vi "User Interface Test.vi"() -> ()   [LabVIEW 2017, in "DSF Core.lvlib"]
uses:
  DSF Core.lvlib
  Typedefs/DSF Version Info.ctl
  Classes/User Interface/Core/Core User Interfaces.lvclass
  C:/Git/DSF/Core/Classes/Component User Interface/Component User Interfaces.lvclass
  Classes/User Interface Handler/User Interface Handler.lvclass
  Classes/User Interface/User Interface.lvclass
  Classes/Component User Interface/Component User Interfaces.lvclass
panel:
  out "settings":cluster{"key":string, "value":string}[](array[cluster])
  in  "stop":bool
  in  "Type":T1(ring)
  out "data format":T2
  in  "stop subpanel":bool
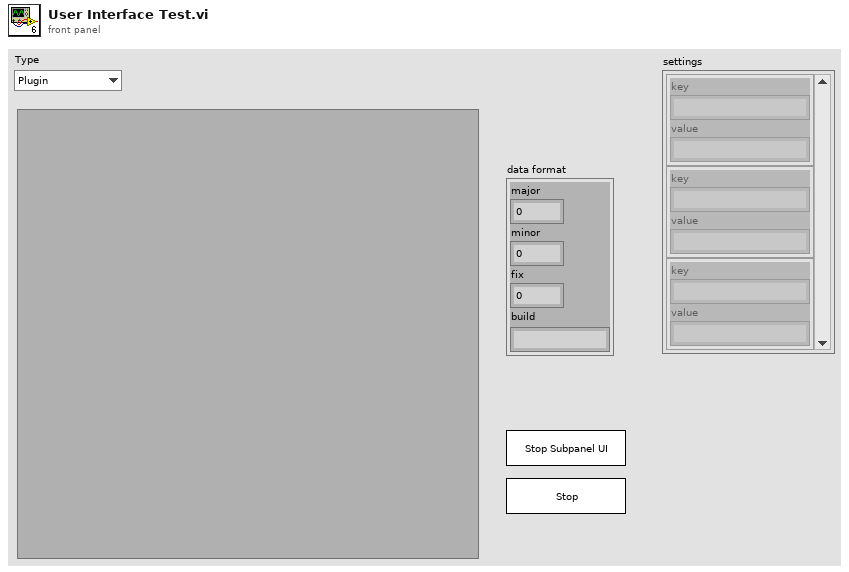
[diagram p1: front panel]
types:
  T1 = enum16{"Plugin", "Thread", "Group", "Transfer", "Channel"}
  T2 = typedef "DSF Core.lvlib/DSF Version Info.ctl" = cluster{"major":u32, "minor":u32, "fix":u32, "build":string}
  T3 = typedef "DSF Core.lvlib/User Interface Handler.lvclass/User Interface Ref.ctl" = refnum<vi>
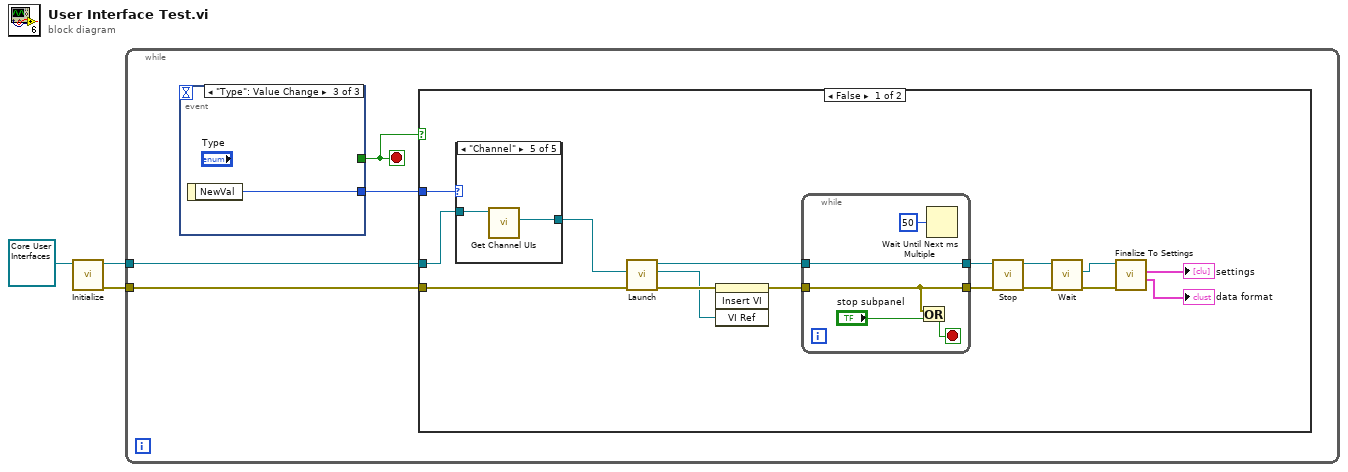
[diagram p0: block diagram]
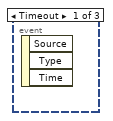
[diagram p2: hidden frame]
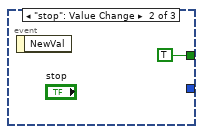
[diagram p3: hidden frame]
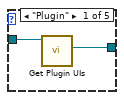
[diagram p4: hidden frame]
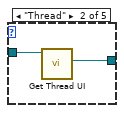
[diagram p5: hidden frame]
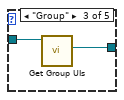
[diagram p6: hidden frame]
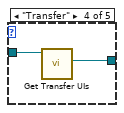
[diagram p7: hidden frame]
diagram:
  n1 = call-dynamic "Initialize.vi"("Component UI in"=refnum<class "Core User Interfaces.lvclass"> refnum ("DSF Core.lvlib:Core Configuration UI.lvclass")) -> ("error out"=w1:errorcluster, "Component UI out"=w2:refnum<class "Core User Interfaces.lvclass">)  [unwired: 9 in]
  n2 = while {
    tunnel: w2 -> [w7]
    tunnel: w1 -> [w4]
    stop <- w6 stop-if-true
    n3 = event shown="[2] \"Type\": Value Change" {
      selector: _ -> [_ _ _]
      dyn-events: _ -> [_ _ _]
      timeout: _ -> [_ _ _]
      tunnel: [_ TRUE _] -> w6
      tunnel: [_ _ w9] -> w5
      event Timeout {
        n4 = event-data() -> ()  [unwired: 1 in, 3 out]
      }
      event "stop": Value Change {
        n5 = event-data() -> ()  [unwired: 1 in, 1 out]
      }
      event "Type": Value Change {
        n6 = event-data() -> ("NewVal"=w9:T1)  [unwired: 1 in]
      }
    }
    n7 = case shown="False" w6 {
      tunnel: w7 -> [w17 _]
      tunnel: w5 -> [w18 _]
      tunnel: w4 -> [w15 _]
      frame False {
        n8 = case shown="\"Channel\"" w18 {
          tunnel: w17 -> [w32 w34 w36 w38 w40]
          tunnel: [w31 w33 w35 w37 w39] -> w11
          frame "Plugin" {
            n9 = call "Get Plugin UIs.vi"("Component UI in"=w32) -> ("Plugin Settings UI"=w31:refnum<class "User Interface.lvclass">)  [unwired: 8 in, 2 out]
          }
          frame "Thread" {
            n10 = call "Get Thread UI.vi"("Component UI in"=w34) -> ("Thread Settings UI"=w33:refnum<class "User Interface.lvclass">)  [unwired: 8 in, 2 out]
          }
          frame "Group" {
            n11 = call "Get Group UIs.vi"("Component UI in"=w36) -> ("Rx Group UI"=w35:refnum<class "User Interface.lvclass">)  [unwired: 7 in, 3 out]
          }
          frame "Transfer" {
            n12 = call "Get Transfer UIs.vi"("Component UI in"=w38) -> ("Rx Transfer UI"=w37:refnum<class "User Interface.lvclass">)  [unwired: 7 in, 3 out]
          }
          frame "Channel" {
            n13 = call "Get Channel UIs.vi"("Component UI in"=w40) -> ("Rx Channel UI"=w39:refnum<class "User Interface.lvclass">)  [unwired: 7 in, 3 out]
          }
        }
        n14 = call "Launch.vi"("error in (no error)"=w15, "User Interface"=w11) -> ("error out"=w14:errorcluster, "active vi"=w13:T3, "User Interface Handler out"=w12:refnum<class "User Interface Handler.lvclass">)  [unwired: 7 in]
        n15 = invoke on="Sub Panel" class="SubPnl" method="Insert VI"(error in=w14, "VI Ref"=w13) -> (error out=w25:errorcluster)  [unwired: 2 in, 3 out]
        n16 = while {
          tunnel: w25 -> [w29]
          tunnel: [w29] -> w23
          tunnel: w12 -> [w26]
          tunnel: [w26] -> w24
          stop <- w27 stop-if-true
          n17 = Or(x=w29, y="stop subpanel") -> (x .or. y?=w27:bool)
          n18 = Wait Until Next ms Multiple(millisecond multiple=u32 50) -> ()  [unwired: 1 out]
        }
        n19 = call "Stop.vi"("error in (no error)"=w23, "User Interface Handler in"=w24) -> ("error out"=w21:errorcluster, "User Interface Handler out"=w22:refnum<class "User Interface Handler.lvclass">)  [unwired: 8 in]
        n20 = call "Wait.vi"("error in (no error)"=w21, "User Interface Handler in"=w22) -> ("error out"=w20:errorcluster, "User Interface"=w10:refnum<class "User Interface.lvclass">)  [unwired: 7 in, 1 out]
        n21 = call "Finalize To Settings.vi"("error in (no error)"=w20, "User Interface in"=w10) -> ("settings version"=→"data format":T2, "settings"=→"settings":cluster{"key":string, "value":string}[])  [unwired: 6 in, 2 out]
      }
      frame True {
      }
    }
  }
